vi "Default Path.vi"(8 "error in (no error)":errorcluster, 11 "client in":refnum<class "Direct SFTP Connection.lvclass">) -> (0 "error out":errorcluster, 2 "path":path, 3 "client out":refnum<class "Direct SFTP Connection.lvclass">)   [LabVIEW 2020, in "NI_SFTP.lvlib" / "Direct SFTP Connection.lvclass"]
uses:
  <vilib>/net/SFTP/Direct SFTP Connection/Direct SFTP Connection.lvclass
  <vilib>/Utility/error.llb/Error Cluster From Error Code.vi
  <vilib>/ErrorRing/Error Ring.xnode
panel:
  out "found?":bool
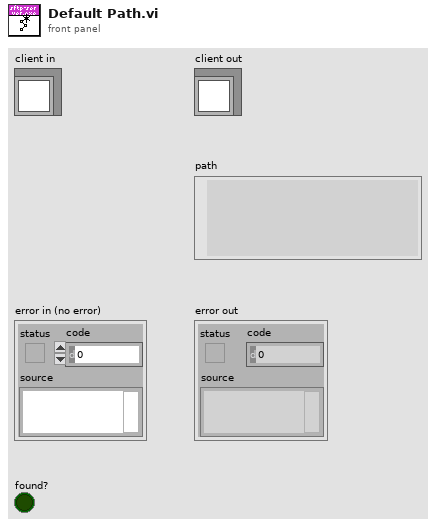
[diagram p1: front panel]
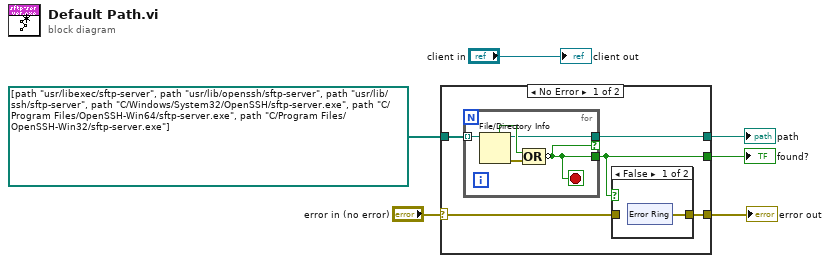
[diagram p0: block diagram]
diagram:
  n1 = case shown="No Error" "error in (no error)" {
    selector: "error in (no error)" -> [w8 w23]
    tunnel: [w7 w23] -> w2
    tunnel: [w9 _] -> w1
    tunnel: [w10 _] -> w4
    tunnel: path[] [path "/usr/libexec/sftp-server", path "/usr/lib/openssh/sftp-server", path "/usr/lib/ssh/sftp-server", path "C:/Windows/System32/OpenSSH/sftp-server.exe", path "C:/Program Files/OpenSSH-Win64/sftp-server.exe", path "C:/Program Files/OpenSSH-Win32/sftp-server.exe"] -> [w11 _]
    frame No Error {
      n2 = for {
        tunnel: w11 -> [w22] mode=indexing
        tunnel: [w18] -> w9
        tunnel: [w19] -> w10 if=w18
        stop <- w18 stop-if-true
        n3 = File/Directory Info(path=w22) -> (path out=w19:path, directory=w20:bool, error out=w21:errorcluster)  [unwired: 1 in, 4 out]
        n4 = Compound Arithmetic op=OR(w20, w21) -> (invert w18:bool)
      }
      n5 = case shown="False" w9 {
        tunnel: w8 -> [_ w17]
        tunnel: [w12 w17] -> w7
        frame False {
          n6 = xnode "Error Ring"() -> ("error out"=w12:errorcluster)
        }
        frame True {
        }
      }
    }
    frame Error {
    }
  }
  "error out" <- w2
  "path" <- w4
  "found?" <- w1
  "client out" <- "client in"
